vi "Move_Completed.vi"(0 "serial master instance":refnum<class "Modbus Master.lvclass">, 11 "error in":errorcluster) -> (4 "Modbus master out":refnum<class "Modbus Master.lvclass">, 6 "Z completed":bool, 8 "Y completed":bool, 10 "X completed":bool, 15 "error out":errorcluster)   [LabVIEW 2018]
uses:
  <vilib>/NI/Modbus Library/API/Master/Modbus Master.lvclass
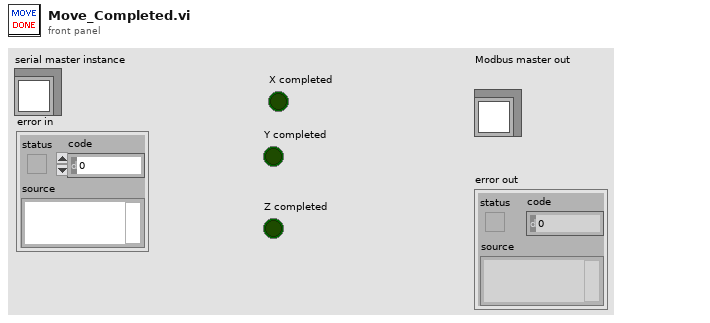
[diagram p1: front panel]
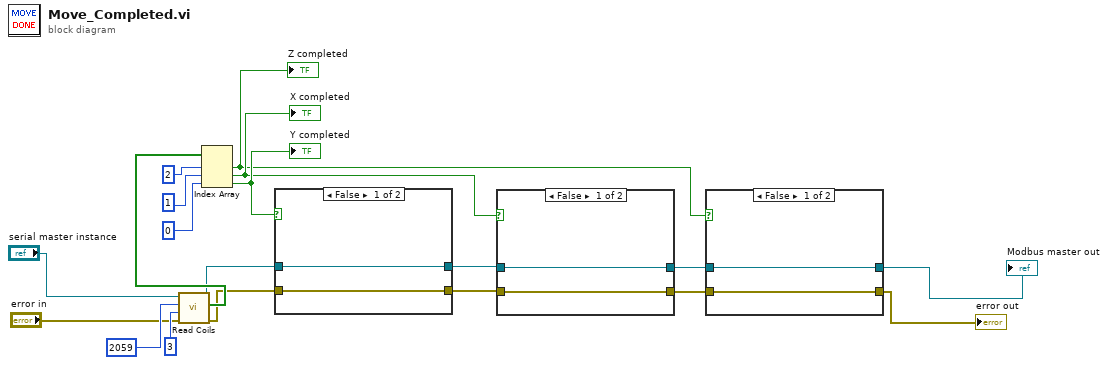
[diagram p0: block diagram]
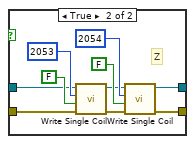
[diagram p2: hidden frame]
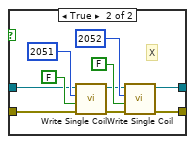
[diagram p3: hidden frame]
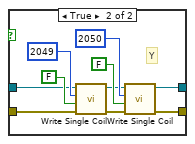
[diagram p4: hidden frame]
diagram:
  n1 = call-dynamic "Read Coils.vi"("error in"="error in", "number of inputs"=u16 3, "starting address"=u16 2059, "Modbus master in"="serial master instance") -> ("error out"=w7:errorcluster, "coils"=w11:bool[], "Modbus master out"=w8:refnum<class "Modbus Master.lvclass">)  [unwired: 5 in]
  n2 = Index Array(array=w11, index #1=2 ("index"), index #2=1 ("index"), index #3=0 ("index")) -> (element #1=w1:bool, element #2=w2:bool, element #3=w3:bool)
  "X completed" <- w2
  "Y completed" <- w3
  "Z completed" <- w1
  n3 = case shown="False" w3 {
    tunnel: w8 -> [w20 w29]
    tunnel: w7 -> [w21 w28]
    tunnel: [w21 w24] -> w15
    tunnel: [w20 w23] -> w16
    frame False {
    }
    frame True {
      # "Y"
      n4 = call-dynamic "Write Single Coil.vi"("error in"=w28, "coil to write"=FALSE, "address"=u16 2049, "Modbus master in"=w29) -> ("error out"=w25:errorcluster, "Modbus master out"=w22:refnum<class "Modbus Master.lvclass">)  [unwired: 6 in]
      n5 = call-dynamic "Write Single Coil.vi"("error in"=w25, "coil to write"=FALSE, "address"=u16 2050, "Modbus master in"=w22) -> ("error out"=w24:errorcluster, "Modbus master out"=w23:refnum<class "Modbus Master.lvclass">)  [unwired: 6 in]
    }
  }
  n6 = case shown="False" w2 {
    tunnel: w16 -> [w32 w41]
    tunnel: w15 -> [w33 w40]
    tunnel: [w33 w36] -> w13
    tunnel: [w32 w35] -> w14
    frame False {
    }
    frame True {
      # "X"
      n7 = call-dynamic "Write Single Coil.vi"("error in"=w40, "coil to write"=FALSE, "address"=u16 2051, "Modbus master in"=w41) -> ("error out"=w37:errorcluster, "Modbus master out"=w34:refnum<class "Modbus Master.lvclass">)  [unwired: 6 in]
      n8 = call-dynamic "Write Single Coil.vi"("error in"=w37, "coil to write"=FALSE, "address"=u16 2052, "Modbus master in"=w34) -> ("error out"=w36:errorcluster, "Modbus master out"=w35:refnum<class "Modbus Master.lvclass">)  [unwired: 6 in]
    }
  }
  n9 = case shown="False" w1 {
    tunnel: w14 -> [w44 w53]
    tunnel: w13 -> [w45 w52]
    tunnel: [w45 w48] -> w4
    tunnel: [w44 w47] -> w12
    frame False {
    }
    frame True {
      # "Z"
      n10 = call-dynamic "Write Single Coil.vi"("error in"=w52, "coil to write"=FALSE, "address"=u16 2053, "Modbus master in"=w53) -> ("error out"=w49:errorcluster, "Modbus master out"=w46:refnum<class "Modbus Master.lvclass">)  [unwired: 6 in]
      n11 = call-dynamic "Write Single Coil.vi"("error in"=w49, "coil to write"=FALSE, "address"=u16 2054, "Modbus master in"=w46) -> ("error out"=w48:errorcluster, "Modbus master out"=w47:refnum<class "Modbus Master.lvclass">)  [unwired: 6 in]
    }
  }
  "error out" <- w4
  "Modbus master out" <- w12
